vi "Flatten Value.vi"(0 "Bool In":refnum<class "Bool.lvclass">, 11 "Error In":errorcluster) -> (4 "Bool Out":refnum<class "Bool.lvclass">, 8 "Value":string, 15 "Error Out":errorcluster)   [LabVIEW 2016, in "Bool.lvclass"]
uses:
  Bool.lvclass
  Bool.lvclass/Bool.ctl
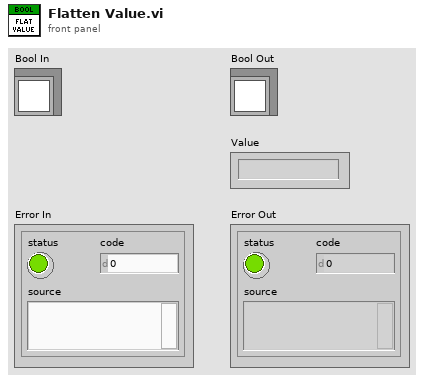
[diagram p1: front panel]
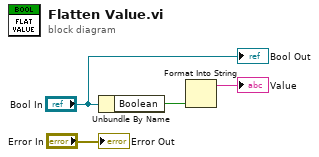
[diagram p0: block diagram]
diagram:
  n1 = Unbundle By Name("Bool In") -> ("Boolean"=w3:bool)
  n2 = Format Into String(w3) -> (resulting string=→"Value":string)  [unwired: 3 in, 1 out]
  "Bool Out" <- "Bool In"
  "Error Out" <- "Error In"
